vi "多反-Overlay槽检出信息.vi"() -> ()   [LabVIEW 2018]
uses:
  <vilib>/vision/Image Controls.llb/IMAQ Image.ctl
panel:
  out "ImgRaw 2":T1
  in  "ImgRaw":T1
  in  "槽检出信息":T2(array[cluster])
  in  "显示槽信息":bool
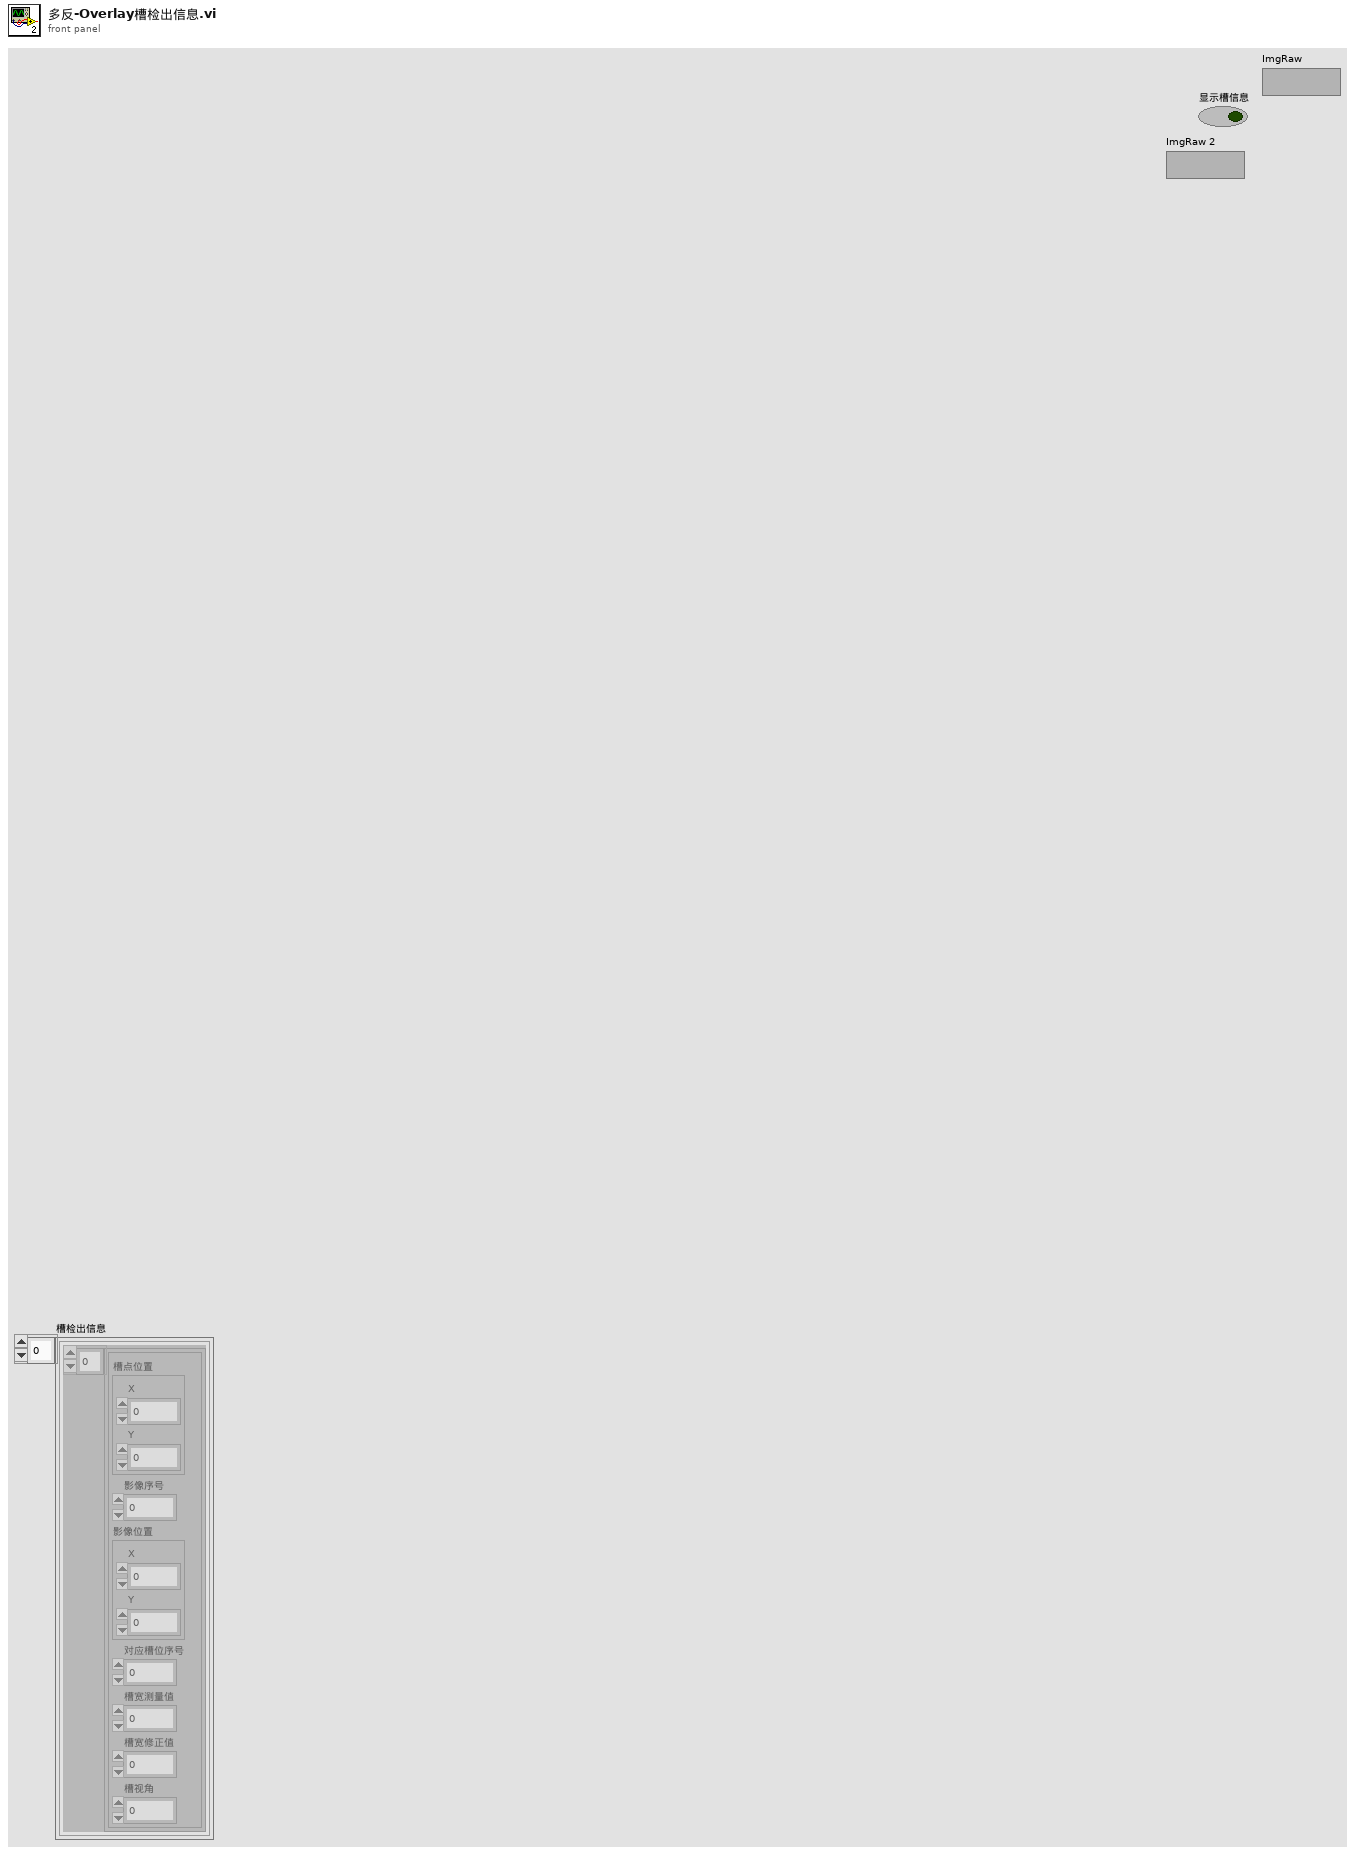
[diagram p1: front panel]
types:
  T1 = typedef "IMAQ Image.ctl" = refnum<image>
  T2 = cluster{cluster{"槽点位置":cluster{"X":sgl, "Y":sgl}, "影像序号":i32, "影像位置":cluster{"X":sgl, "Y":sgl}, "对应槽位序号":i32, "槽宽测量值":dbl, "槽宽修正值":dbl, "槽视角":dbl}[]}[]
  T3 = cluster{"槽点位置":cluster{"X":sgl, "Y":sgl}, "影像序号":i32, "影像位置":cluster{"X":sgl, "Y":sgl}, "对应槽位序号":i32, "槽宽测量值":dbl, "槽宽修正值":dbl, "槽视角":dbl}[]
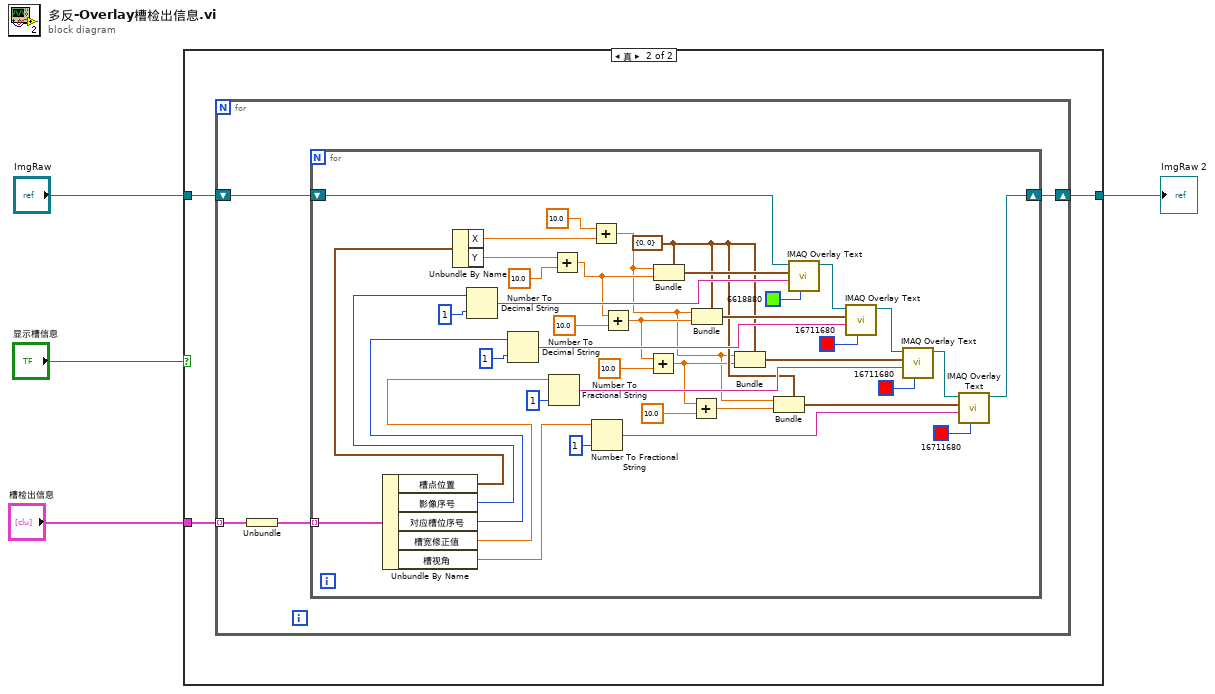
[diagram p0: block diagram]
diagram:
  n1 = case shown="真" "显示槽信息" {
    tunnel: "槽检出信息" -> [_ w8]
    tunnel: "ImgRaw" -> [w5 w7]
    tunnel: [w5 w6] -> w1
    frame False {
    }
    frame True {
      n2 = for {
        tunnel: w8 -> [w10] mode=indexing
        shift-right: [w11] -> w6
        shift-left: w7 -> [w12]
        n3 = Unbundle(w10) -> (w9:T3)
        n4 = for {
          tunnel: w9 -> [w13] mode=indexing
          shift-right: [w20] -> w11
          shift-left: w12 -> [w21]
          w28 = cluster{"X":i32, "Y":i32} {"X"=0, "Y"=0} ("Origin")
          n5 = Unbundle By Name(w13) -> ("槽点位置"=w26:cluster{"X":sgl, "Y":sgl}, "影像序号"=w25:i32, "对应槽位序号"=w24:i32, "槽宽修正值"=w23:dbl, "槽视角"=w22:dbl)
          n6 = Unbundle By Name(w26) -> ("X"=w14:sgl, "Y"=w18:sgl)
          n7 = Number To Decimal String(number=w25, width (-)=i16 1 ("精度(6)")) -> (decimal integer string=w51:string)
          n8 = Number To Decimal String(number=w24, width (-)=i16 1 ("精度(6)")) -> (decimal integer string=w42:string)
          n9 = Number To Fractional String(number=w23, precision (6)=i16 1 ("精度(6)")) -> (F-format string=w41:string)  [unwired: 2 in]
          n10 = Add(x=w18, y=10.0) -> (x+y=w16:dbl)
          n11 = Add(x=10.0 ("y"), y=w14) -> (x+y=w15:dbl)
          n12 = Number To Fractional String(number=w22, precision (6)=i16 1 ("精度(6)")) -> (F-format string=w32:string)  [unwired: 2 in]
          n13 = Add(x=w16, y=10.0) -> (x+y=w36:dbl)
          n14 = Add(x=w36, y=10.0) -> (x+y=w27:dbl)
          n15 = Bundle(cluster=w28, "X"=w15, "Y"=w16) -> (w52:cluster{"X":i32, "Y":i32})
          n16 = Add(x=w27, y=10.0) -> (x+y=w34:dbl)
          n17 = Bundle(cluster=w28, "X"=w15, "Y"=w36) -> (w40:cluster{"X":i32, "Y":i32})
          n18 = Bundle(cluster=w28, "X"=w15, "Y"=w27) -> (w37:cluster{"X":i32, "Y":i32})
          n19 = Bundle(cluster=w28, "X"=w15, "Y"=w34) -> (w35:cluster{"X":i32, "Y":i32})
          n20 = call "IMAQ Overlay Text"("Text Color (black)"=u32 6618880, "String"=w51, "Origin"=w52, "Image"=w21) -> ("Image Out"=w44:T1)  [unwired: 6 in, 1 out]
          n21 = call "IMAQ Overlay Text"("Text Color (black)"=u32 16711680, "String"=w42, "Origin"=w40, "Image"=w44) -> ("Image Out"=w43:T1)  [unwired: 6 in, 1 out]
          n22 = call "IMAQ Overlay Text"("Text Color (black)"=u32 16711680, "String"=w41, "Origin"=w37, "Image"=w43) -> ("Image Out"=w29:T1)  [unwired: 6 in, 1 out]
          n23 = call "IMAQ Overlay Text"("Text Color (black)"=u32 16711680, "String"=w32, "Origin"=w35, "Image"=w29) -> ("Image Out"=w20:T1)  [unwired: 6 in, 1 out]
        }
      }
    }
  }
  "ImgRaw 2" <- w1
